vi "CreateDMAtask.vi"(0 "Accele Task":T2={"Accele Task"=[], "Simulate"=FALSE, "采样率"={"AISampleRate"=10123, "CouplingType"=10000, "Butter"=1000}, "Trig"={"PreTrigCNT"=0, "TriggerMode"=enum."中间触发", "TriggerSource"=enum."软件触发", "ATRTriggerChannel"=enum."通道0", "TriggerDir"=enum."下降沿触发", "TrigLevelVolt"=0.0, "bAvailableTrig"=FALSE}, "clock"={"EN"=FALSE, "clocksource"=enum."内部时钟", "outclocksource"=enum."Trig0"}, "delay(S)"=0.0} {"采样率"."CouplingType" items=["直流耦合", "交流耦合"]}, 3 "error in (no error)":errorcluster) -> (7 "task":T1={"Task Info"={"Accele Task"=[], "Simulate"=FALSE, "采样率"={"AISampleRate"=10123, "CouplingType"=10000, "Butter"=1000}, "Trig"={"PreTrigCNT"=0, "TriggerMode"=enum."中间触发", "TriggerSource"=enum."软件触发", "ATRTriggerChannel"=enum."通道0", "TriggerDir"=enum."下降沿触发", "TrigLevelVolt"=0.0, "bAvailableTrig"=FALSE}, "clock"={"EN"=FALSE, "clocksource"=enum."内部时钟", "outclocksource"=enum."Trig0"}, "delay(S)"=0.0}, "datain"={"nSegmentCount"=0, "chaneldataSize"=8192, "t0 in"=timestamp(0 s since 1904-01-01), "nsegmentsize"=0, "chanelcouter"=0}, "times"=0.0, "timer"=[], "\nen"=FALSE} {"Task Info"."采样率"."CouplingType" items=["直流耦合", "交流耦合"]}, 10 "error out":errorcluster)   [LabVIEW 2009]
uses:
  Ctrls/Device.ctl
  Ctrls/Acceleration Channel Config_Ctrls-某型振动实验台测试系统.ctl
  Ctrls/Sample Information.ctl
  Ctrls/Trig.ctl
  Ctrls/clock.ctl
  Ctrls/Task Info.ctl
  Ctrls/task.ctl
  Ctrls/DATA info.ctl
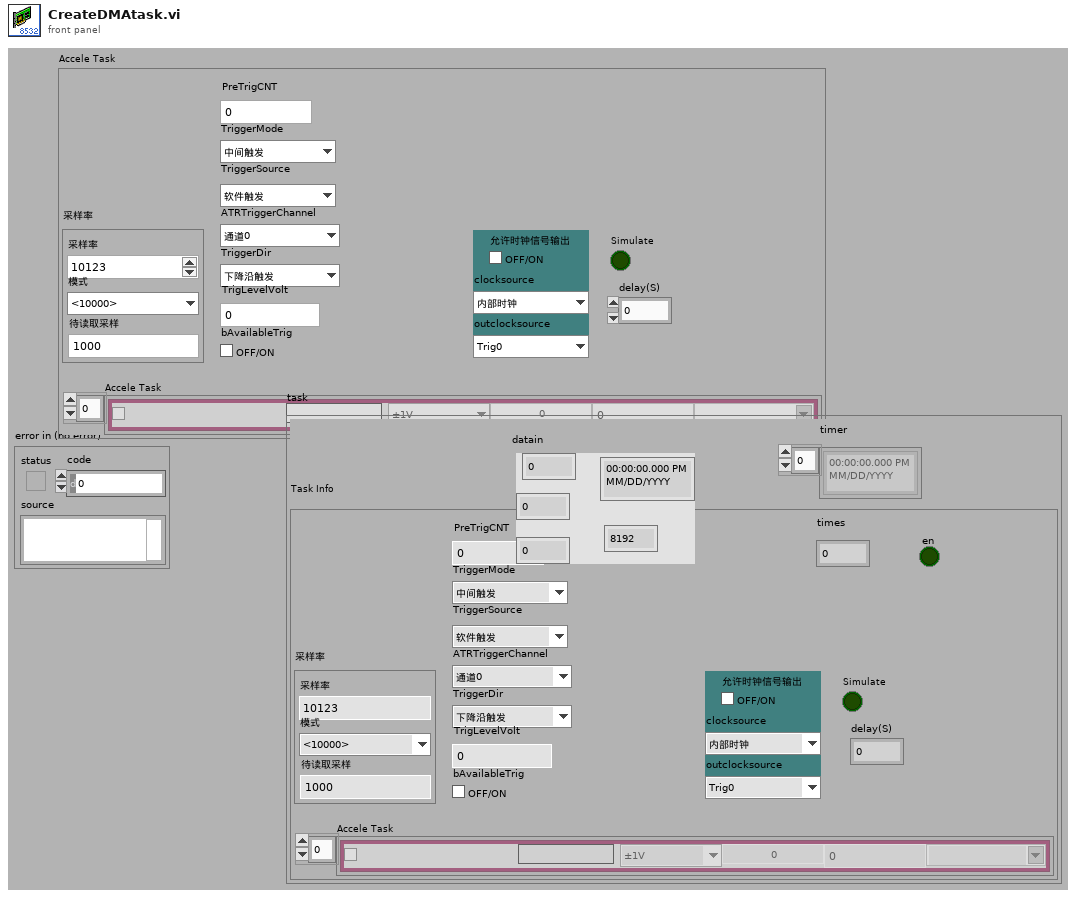
[diagram p1: front panel]
types:
  T1 = typedef "task.ctl" = cluster{"Task Info":T2, "datain":T7, "times":dbl, "timer":timestamp[], "\nen":bool}
  T2 = typedef "Task Info.ctl" = cluster{"Accele Task":T3[], "Simulate":bool, "采样率":T4, "Trig":T5, "clock":T6, "delay(S)":dbl}
  T3 = typedef "Acceleration Channel Config_Ctrls-某型振动实验台测试系统.ctl" = cluster{"Enable":bool, "Name":string, "range":enum16{"±1V", "±5V"}, "SensValue":dbl, "PhysicalName":string, "off":dbl, "Sensunits":string}
  T4 = typedef "Sample Information.ctl" = cluster{"AISampleRate":i32, "CouplingType":i32, "Butter":i32}
  T5 = typedef "Trig.ctl" = cluster{"PreTrigCNT":i32, "TriggerMode":enum16{"中间触发", "后触发", "预触发", "硬件延时触发"}, "TriggerSource":enum16{"软件触发", "DTR信号源", "ATR信号源", "Triger信号触发"}, "ATRTriggerChannel":enum16{"通道0", "通道1", "通道2", "通道3"}, "TriggerDir":enum16{"下降沿触发", "上升沿触发", "上下边没均触发"}, "TrigLevelVolt":sgl, "bAvailableTrig":bool}
  T6 = typedef "clock.ctl" = cluster{"EN":bool, "clocksource":enum16{"内部时钟", "外部时钟"}, "outclocksource":enum16{"Trig0", "Trig1", "Trig2", "Trig3", "Trig4", "Trig5", "Trig6", "Trig7", "PXI_STAR"}}
  T7 = typedef "DATA info.ctl" = cluster{"nSegmentCount":i32, "chaneldataSize":i32, "t0 in":timestamp, "nsegmentsize":i32, "chanelcouter":i32}
  T8 = typedef "Device.ctl" = cluster{"hDevice":i32, "hDmaEvent":i32}
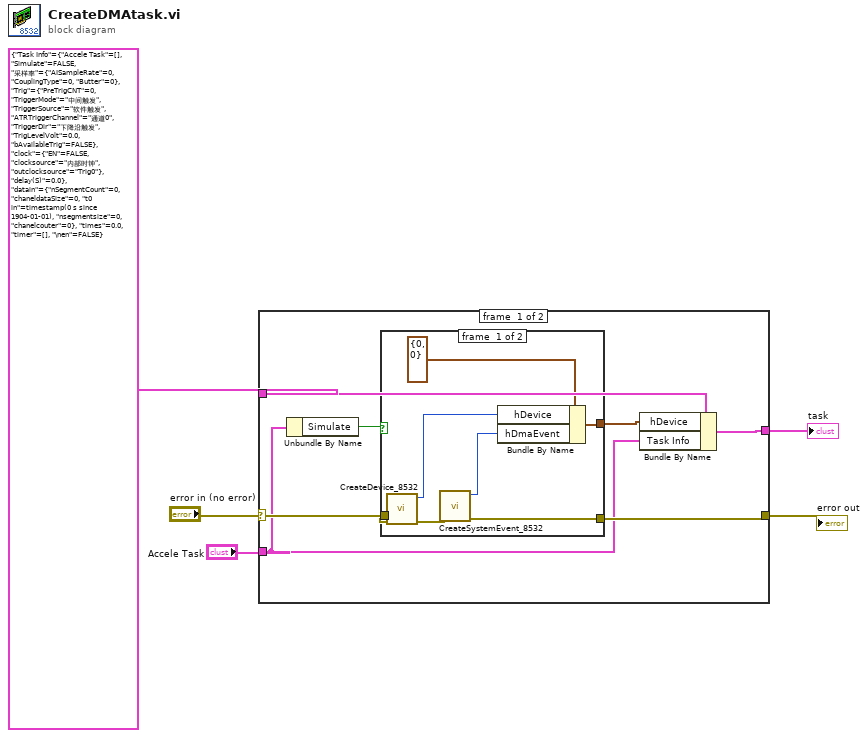
[diagram p0: block diagram]
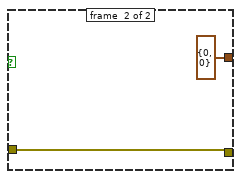
[diagram p2: hidden frame]
diagram:
  n1 = case shown="无错误" "error in (no error)" {
    selector: "error in (no error)" -> [w8 w23]
    tunnel: [w12 w23] -> w4
    tunnel: "Accele Task" -> [w7 _]
    tunnel: T1 {"Task Info"={"Accele Task"=[], "Simulate"=FALSE, "采样率"={"AISampleRate"=0, "CouplingType"=0, "Butter"=0}, "Trig"={"PreTrigCNT"=0, "TriggerMode"=enum."中间触发", "TriggerSource"=enum."软件触发", "ATRTriggerChannel"=enum."通道0", "TriggerDir"=enum."下降沿触发", "TrigLevelVolt"=0.0, "bAvailableTrig"=FALSE}, "clock"={"EN"=FALSE, "clocksource"=enum."内部时钟", "outclocksource"=enum."Trig0"}, "delay(S)"=0.0}, "datain"={"nSegmentCount"=0, "chaneldataSize"=0, "t0 in"=timestamp(0 s since 1904-01-01), "nsegmentsize"=0, "chanelcouter"=0}, "times"=0.0, "timer"=[], "\nen"=FALSE} ("task") -> [w10 w22]
    tunnel: [w11 w22] -> w3
    frame #0 {
      n2 = Unbundle By Name(w7) -> ("Simulate"=w6:bool)
      n3 = case shown="假" w6 {
        tunnel: [w19 w20] -> w12
        tunnel: [w16 T8 {"hDevice"=0, "hDmaEvent"=0} ("hDevice")] -> w9
        tunnel: w8 -> [w14 w20]
        frame #0 {
          n4 = call "CreateDevice_8532.vi"("error in (no error)"=w14) -> ("error out"=w15:errorcluster, "hDevice"=w13:i32)  [unwired: 9 out]
          n5 = call "CreateSystemEvent_8532.vi"("error in (no error)"=w15) -> ("error out"=w19:errorcluster, "hEvent"=w17:i32)  [unwired: 9 out]
          n6 = Bundle By Name(cluster=T8 {"hDevice"=0, "hDmaEvent"=0} ("hDevice"), "hDevice"=w13, "hDmaEvent"=w17) -> (w16:T8)
        }
        frame #1 {
        }
      }
      n7 = Bundle By Name(cluster=w10, "hDevice"=w9, "Task Info"=w7) -> (w11:T1)
    }
    frame #1 {
    }
  }
  "error out" <- w4
  "task" <- w3
